vi "Log.Warning.vi"(8 "error in":errorcluster, 9 "Append newline? (T)":bool=TRUE, 10 "Add to log file? (F)":bool, 11 "Message":string) -> (0 "error out":errorcluster)   [LabVIEW 2026, in "NIDMM Engine.lvlib" / "NIDMM Engine.lvclass"]
uses:
  NIDMM Engine.lvclass
  NIDMM Engine.lvclass/NIDMM Engine.ctl
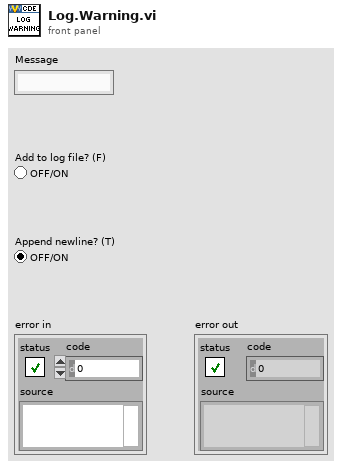
[diagram p1: front panel]
types:
  T1 = cluster{"Message":string, "Level":enum16{"Error", "Warning", "Info", "Debug"}, "Add to log file? (F)":bool, "Append newline? (T)":bool}
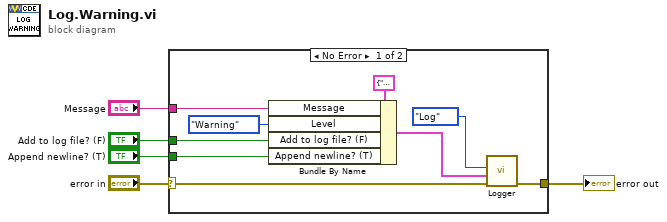
[diagram p0: block diagram]
diagram:
  n1 = case shown="No Error" "error in" {
    selector: "error in" -> [w14 w15]
    tunnel: "Message" -> [w11 _]
    tunnel: "Add to log file? (F)" -> [w9 _]
    tunnel: "Append newline? (T)" -> [w8 _]
    tunnel: [w13 w15] -> w4
    frame No Error {
      n2 = Bundle By Name(cluster=T1 {"Message"="", "Level"=enum."Error", "Add to log file? (F)"=FALSE, "Append newline? (T)"=TRUE} ("Log"), "Message"=w11, "Level"=enum16{"Error", "Warning", "Info", "Debug"}."Warning", "Add to log file? (F)"=w9, "Append newline? (T)"=w8) -> (w6:T1)
      n3 = call "Logger.vi"("error in"=w14, "Log"=w6, "State"=enum16{"Initialize", "Log"}."Log") -> ("error out"=w13:errorcluster)  [unwired: 7 in, 1 out]
    }
    frame Error {
    }
  }
  "error out" <- w4
